vi "Inst.KH7008.handleSetCommand.vi"(8 "error in (no error)":errorcluster, 9 "Data":variant, 10 "Command":string, 11 "Inst.Krohn-Hite-7008 in":refnum<class "Inst.Krohn-Hite-7008.lvclass">) -> (0 "error out":errorcluster, 3 "Inst.Krohn-Hite-7008 out":refnum<class "Inst.Krohn-Hite-7008.lvclass">)   [LabVIEW 2019, in "Inst.KH7008.lvlib" / "Inst.Krohn-Hite-7008.lvclass"]
uses:
  Inst.Krohn-Hite-7008.lvclass
  Inst.Krohn-Hite-7008.lvclass/Inst.Krohn-Hite-7008.ctl
  Typedefs/setAllChannelsRequest--Cluster.ctl
  KH7008/typedefs/allChannelProperties--Array.ctl
  KH7008/typedefs/channelProperties--Cluster.ctl
  KH7008/typedefs/channel--numeric.ctl
  KH7008/typedefs/gain--enum.ctl
  KH7008/typedefs/Input--Enum.ctl
  KH7008/typedefs/shunt--enum.ctl
  KH7008/typedefs/couple--Enum.ctl
  KH7008/typedefs/Filter--Enum.ctl
  ccddaa8b-c58a-444d-bab3-be5a42c0077d.vi
  ccddaa8b-c58a-444d-bab3-be5a42c0077d.vi/6595d90c-c030-4b34-929f-62487217dac0.vi
  ccddaa8b-c58a-444d-bab3-be5a42c0077d.vi/01b853ae-85f8-4b3f-90b0-c5197e57e7e2.vi
  <vilib>/Utility/Data Type/Get Type Information.vi
  <vilib>/JDP Science/JSONtext/JSON text to Variant.vi
  <vilib>/JDP Science/JSONtext/LVClass Serializer/JSONtext LVClass Serializer.lvclass
  KH7008/KH7008.lvlib
  <vilib>/JDP Science/JSONtext/JSONtext.lvlib
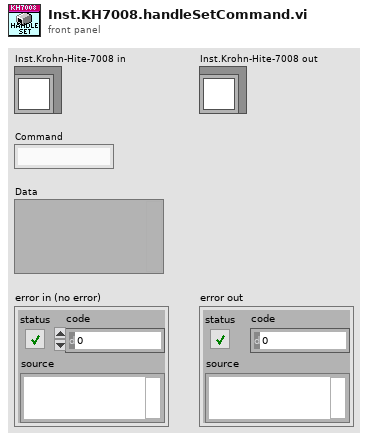
[diagram p1: front panel]
types:
  T1 = typedef "Inst.KH7008.lvlib/Inst.Krohn-Hite-7008.lvclass/setAllChannelsRequest--Cluster.ctl" = cluster{"allChannelProperties":T2}
  T2 = typedef "KH7008.lvlib/allChannelProperties--Array.ctl" = T3[]
  T3 = typedef "KH7008.lvlib/channelProperties--Cluster.ctl" = cluster{"channel":T4, "gain":T5, "input":T6, "shunt":T7, "couple":T8, "filter":T9}
  T4 = typedef "KH7008.lvlib/channel--numeric.ctl" = u16
  T5 = typedef "KH7008.lvlib/gain--enum.ctl" = enum16{"1", "10", "100", "1000"}
  T6 = typedef "KH7008.lvlib/Input--Enum.ctl" = enum16{"OFF", "SE+", "SE-", "DIFF"}
  T7 = typedef "KH7008.lvlib/shunt--enum.ctl" = enum16{"Open", "50", "500", "5k", "50k", "10M"}
  T8 = typedef "KH7008.lvlib/couple--Enum.ctl" = enum16{"AC", "DC"}
  T9 = typedef "KH7008.lvlib/Filter--Enum.ctl" = enum16{"OFF", "ON"}
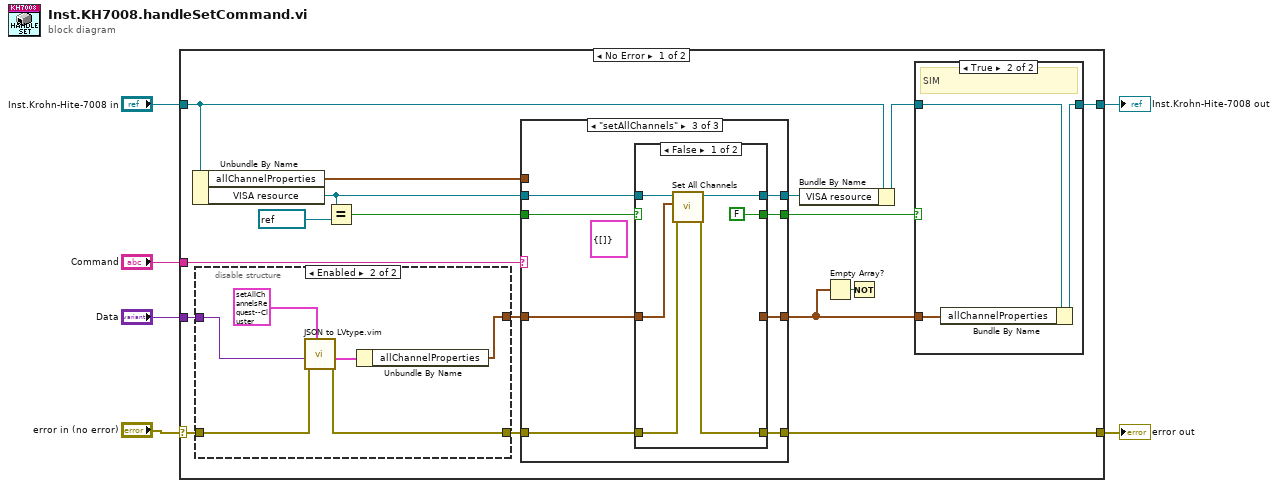
[diagram p0: block diagram]
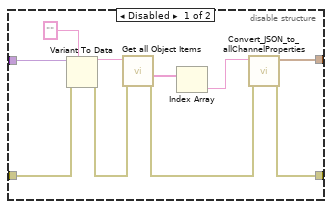
[diagram p2: hidden frame]
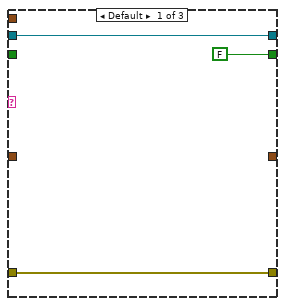
[diagram p3: hidden frame]
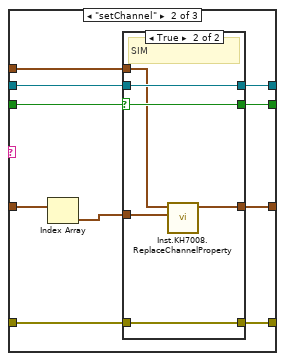
[diagram p4: hidden frame]
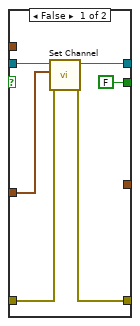
[diagram p5: hidden frame]
diagram:
  n1 = case shown="No Error" "error in (no error)" {
    selector: "error in (no error)" -> [w9 w87]
    tunnel: "Command" -> [w23 _]
    tunnel: "Data" -> [w10 _]
    tunnel: [w17 w88] -> w3
    tunnel: "Inst.Krohn-Hite-7008 in" -> [w22 w88]
    tunnel: [w21 w87] -> w1
    frame No Error {
      n2 = Unbundle By Name(w22) -> ("allChannelProperties"=w12:T2, "VISA resource"=w19:refnum<visa-resource-name>)
      n3 = disable-structure shown="Enabled" {
        disable-tunnel: w10 -> [w30 w38]
        disable-tunnel: w9 -> [w28 w37]
        disable-tunnel: [w27 w36] -> w8
        disable-tunnel: [w24 w34] -> w7
        frame Disabled {
          n4 = Variant To Data(error in=w28, type="", Variant=w30) -> (data=w31:string, error out=w25:errorcluster)
          n5 = call <vilib>:"Get all Object Items.vi"("error in (no error)"=w25, "JSON"=w31) -> ("error out"=w26:errorcluster, "<JSON>"=w33:string[])  [unwired: 6 in, 2 out]
          n6 = Index Array(array=w33) -> (element=w32:string)  [unwired: 1 in]
          n7 = call "Convert_JSON_to_allChannelProperties.vi"("error in (no error)"=w26, "<JSON>"=w32) -> ("error out"=w27:errorcluster, "allChannelProperties"=w24:T2)  [unwired: 8 in]
        }
        frame Enabled {
          n8 = call "JSON to LVtype.vim"("type"=T1 {"allChannelProperties"=[{"channel"=1, "gain"=enum."10", "input"=enum."OFF", "shunt"=enum."10M", "couple"=enum."AC", "filter"=enum."OFF"}, {"channel"=2, "gain"=enum."10", "input"=enum."OFF", "shunt"=enum."10M", "couple"=enum."AC", "filter"=enum."OFF"}, {"channel"=3, "gain"=enum."10", "input"=enum."OFF", "shunt"=enum."10M", "couple"=enum."AC", "filter"=enum."OFF"}, {"channel"=4, "gain"=enum."10", "input"=enum."OFF", "shunt"=enum."10M", "couple"=enum."AC", "filter"=enum."OFF"}, {"channel"=5, "gain"=enum."10", "input"=enum."OFF", "shunt"=enum."10M", "couple"=enum."AC", "filter"=enum."OFF"}, {"channel"=6, "gain"=enum."10", "input"=enum."OFF", "shunt"=enum."10M", "couple"=enum."AC", "filter"=enum."OFF"}, {"channel"=7, "gain"=enum."10", "input"=enum."OFF", "shunt"=enum."10M", "couple"=enum."AC", "filter"=enum."OFF"}, {"channel"=7, "gain"=enum."10", "input"=enum."OFF", "shunt"=enum."10M", "couple"=enum."AC", "filter"=enum."OFF"}]} ("setAllChannelsRequest"), "error in (no error)"=w37, "JSON Data in"=w38) -> ("error out"=w36:errorcluster, "Data out"=w35:T1)  [unwired: 7 in]
          n9 = Unbundle By Name(w35) -> ("allChannelProperties"=w34:T2)
        }
      }
      n10 = Equal?(x=w19, y=refnum<visa-resource-name> "sim") -> (x = y?=w13:bool)
      n11 = case shown="\"setAllChannels\"" w23 {
        tunnel: w8 -> [w41 w45 w66]
        tunnel: [w42 w52 w72] -> w18
        tunnel: [w41 w51 w71] -> w21
        tunnel: w19 -> [w42 w50 w70]
        tunnel: w13 -> [_ w49 w69]
        tunnel: [_ w46 w68] -> w14
        tunnel: [FALSE w48 w67] -> w11
        tunnel: w12 -> [_ w47 _]
        tunnel: w7 -> [_ w44 w65]
        frame Default {
        }
        frame "setChannel" {
          n12 = Index Array(array=w44) -> (element=w43:T3)  [unwired: 1 in]
          n13 = case shown="True" w49 {
            selector: w49 -> [_ w62]
            tunnel: w45 -> [w58 w63]
            tunnel: [w57 w64] -> w52
            tunnel: [w56 w63] -> w51
            tunnel: w50 -> [w55 w64]
            tunnel: w43 -> [w54 w61]
            tunnel: [FALSE w62] -> w48
            tunnel: w47 -> [_ w59]
            tunnel: [_ w60] -> w46
            frame False {
              n14 = call "Set Channel.vi"("error in (no error)"=w58, "channelParameter"=w54, "VISA Refnum in"=w55) -> ("error out"=w56:errorcluster, "VISA Refnum out"=w57:refnum<visa-resource-name>)  [unwired: 7 in]
            }
            frame True {
              # "SIM"
              n15 = call "Inst.KH7008.ReplaceChannelProperty.vi"("channelProperties"=w61, "allChannelProperties"=w59) -> ("allChannelProperties"=w60:T2)  [unwired: 9 in]
            }
          }
        }
        frame "setAllChannels" {
          (unwired) T1 {"allChannelProperties"=[]} ("setAllChannelRequest")
          n16 = case shown="False" w69 {
            selector: w69 -> [_ w79]
            tunnel: w66 -> [w78 w81]
            tunnel: [w77 w82] -> w72
            tunnel: [w76 w81] -> w71
            tunnel: w70 -> [w75 w82]
            tunnel: w65 -> [w74 w80]
            tunnel: [_ w80] -> w68
            tunnel: [FALSE w79] -> w67
            frame False {
              n17 = call "Set All Channels.vi"("error in (no error)"=w78, "allChannelProperties"=w74, "VISA Refnum in"=w75) -> ("error out"=w76:errorcluster, "VISA Refnum out"=w77:refnum<visa-resource-name>)  [unwired: 6 in, 1 out]
            }
            frame True {
              # "SIM"
            }
          }
        }
      }
      n18 = Bundle By Name(cluster=w22, "VISA resource"=w18) -> (w16:refnum<class "Inst.Krohn-Hite-7008.lvclass">)
      n19 = Empty Array?(array=w14) -> (empty?=w15:bool)
      n20 = Not(x=w15) -> ()  [unwired: 1 out]
      n21 = case shown="True" w11 {
        tunnel: [w83 w86] -> w17
        tunnel: w16 -> [w83 w85]
        tunnel: w14 -> [_ w84]
        frame False {
        }
        frame True {
          # "SIM"
          n22 = Bundle By Name(cluster=w85, "allChannelProperties"=w84) -> (w86:refnum<class "Inst.Krohn-Hite-7008.lvclass">)
        }
      }
    }
    frame Error {
    }
  }
  "Inst.Krohn-Hite-7008 out" <- w3
  "error out" <- w1
